vi "set HovaCAL Sollwerte je MFC.vi"(9 "Messdaten":sgl[](array[numeric]), 10 "MFC in":u32, 11 "Sollwert je MFC Cluster (Eingang)":T1) -> (3 "Sollwert je MFC Cluster (Ausgang)":T1)   [LabVIEW 2020, in "Linearisierung v2.lvlib"]
uses:
  Linearisierung v2.lvlib
  HovaCAL Sollwerte je MFC Cluster.ctl
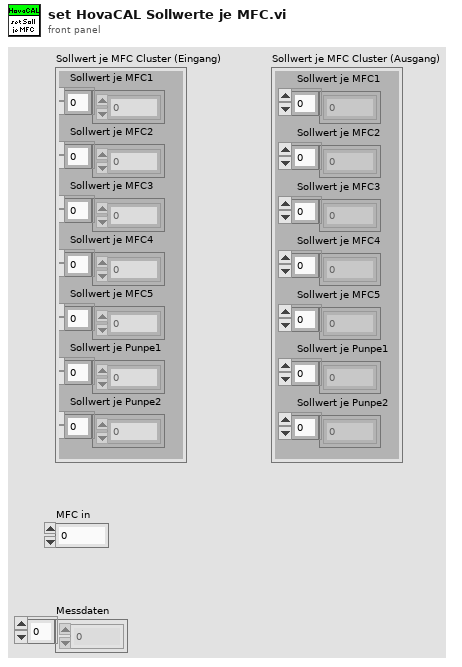
[diagram p1: front panel]
types:
  T1 = typedef "Linearisierung v2.lvlib/HovaCAL Sollwerte je MFC Cluster.ctl" = cluster{"Sollwert je MFC1":sgl[], "Sollwert je MFC2":sgl[], "Sollwert je MFC3":sgl[], "Sollwert je MFC4":sgl[], "Sollwert je MFC5":sgl[], "Sollwert je Punpe1":sgl[], "Sollwert je Punpe2":sgl[]}
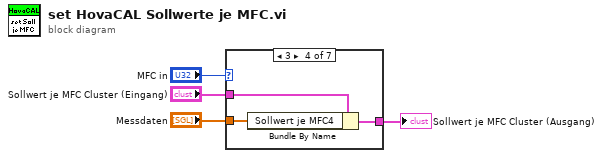
[diagram p0: block diagram]
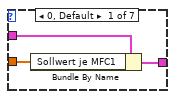
[diagram p2: hidden frame]
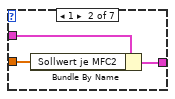
[diagram p3: hidden frame]
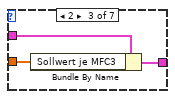
[diagram p4: hidden frame]
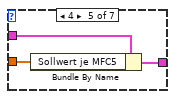
[diagram p5: hidden frame]
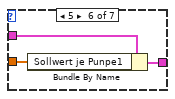
[diagram p6: hidden frame]
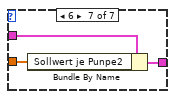
[diagram p7: hidden frame]
diagram:
  n1 = case shown="3" "MFC in" {
    tunnel: "Sollwert je MFC Cluster (Eingang)" -> [w7 w10 w13 w16 w19 w22 w25]
    tunnel: "Messdaten" -> [w6 w9 w12 w15 w18 w21 w24]
    tunnel: [w5 w8 w11 w14 w17 w20 w23] -> w4
    frame 0, Default {
      n2 = Bundle By Name(cluster=w7, "Sollwert je MFC1"=w6) -> (w5:T1)
    }
    frame 1 {
      n3 = Bundle By Name(cluster=w10, "Sollwert je MFC2"=w9) -> (w8:T1)
    }
    frame 2 {
      n4 = Bundle By Name(cluster=w13, "Sollwert je MFC3"=w12) -> (w11:T1)
    }
    frame 3 {
      n5 = Bundle By Name(cluster=w16, "Sollwert je MFC4"=w15) -> (w14:T1)
    }
    frame 4 {
      n6 = Bundle By Name(cluster=w19, "Sollwert je MFC5"=w18) -> (w17:T1)
    }
    frame 5 {
      n7 = Bundle By Name(cluster=w22, "Sollwert je Punpe1"=w21) -> (w20:T1)
    }
    frame 6 {
      n8 = Bundle By Name(cluster=w25, "Sollwert je Punpe2"=w24) -> (w23:T1)
    }
  }
  "Sollwert je MFC Cluster (Ausgang)" <- w4
